vi "Upload Package to SLE.vi"(0 "PACKAGE_PATH":path, 5 "FEED_NAME":string, 11 "error in (no error)":errorcluster) -> (15 "error out":errorcluster)   [LabVIEW 2021, in "Measurement Builder.lvlib"]
uses:
  Measurement Builder.lvlib
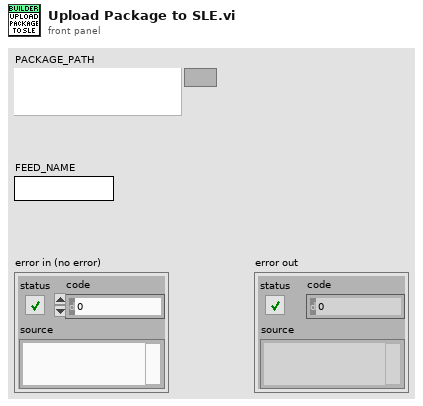
[diagram p1: front panel]
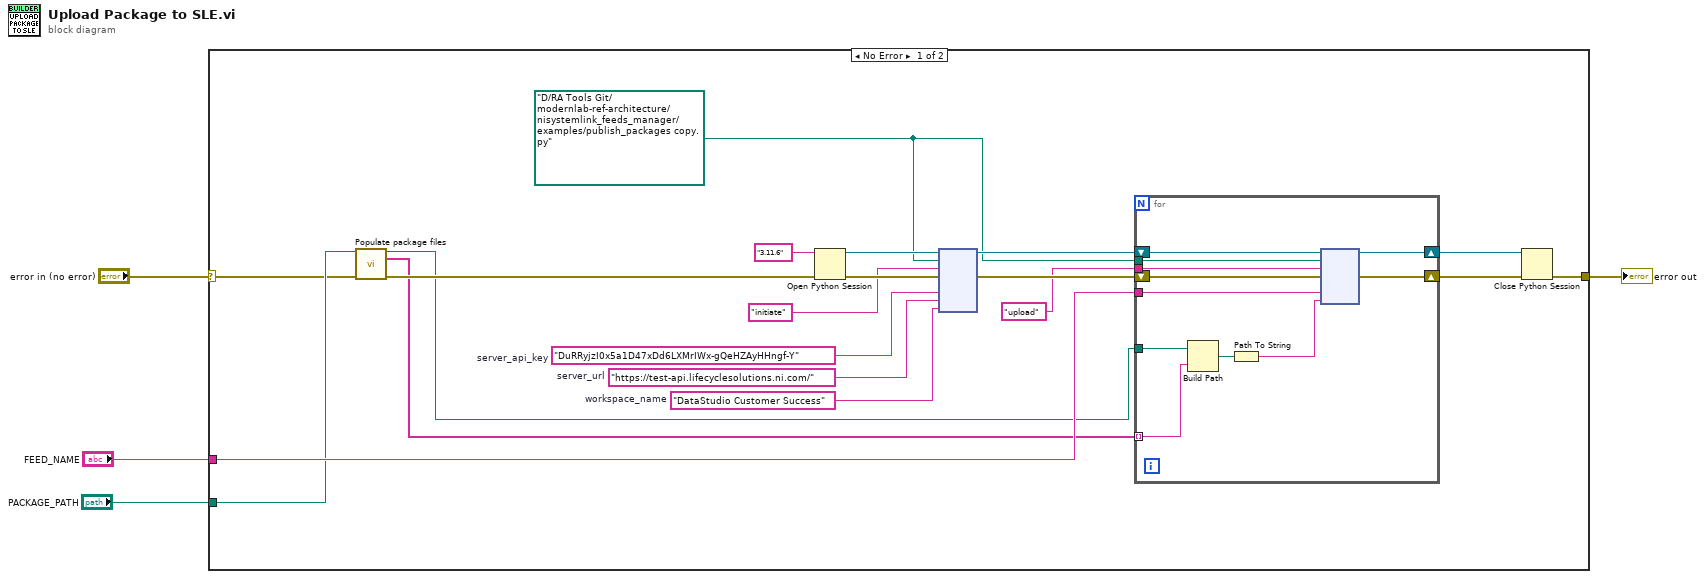
[diagram p0: block diagram]
diagram:
  n1 = case shown="No Error" "error in (no error)" {
    selector: "error in (no error)" -> [w8 w36]
    tunnel: "FEED_NAME" -> [w11 _]
    tunnel: "PACKAGE_PATH" -> [w9 _]
    tunnel: [w10 w36] -> w1
    frame No Error {
      w18 = "DataStudio Customer Success"  # workspace_name
      w19 = "https://test-api.lifecyclesolutions.ni.com/"  # server_url
      w20 = "DuRRyjzI0x5a1D47xDd6LXMrIWx-gQeHZAyHHngf-Y"  # server_api_key
      w12 = path "D:/RA Tools Git/modernlab-ref-architecture/nisystemlink_feeds_manager/examples/publish_packages copy.py" ("module path")
      n2 = call "Populate package files.vi"("Packages Path"=w9, "error in (no error)"=w8) -> ("path out"=w6:path, "filenames"=w5:string[], "error out"=w7:errorcluster)  [unwired: 11 in]
      n3 = Open Python Session(python version="3.11.6" ("Python version"), 3:w7) -> (session out=w23:refnum<k35>, error out=w22:errorcluster)  [unwired: 1 in]
      n4 = node(w23, w12, "initiate" ("function name"), w22, w20, w19, w18) -> (w17:refnum<k35>, w15:errorcluster)  [unwired: 5 in, 2 out]
      n5 = for {
        tunnel: "upload" ("function name") -> [w31]
        tunnel: w12 -> [w30]
        tunnel: w11 -> [w29]
        shift-right: [w34] -> w16
        shift-left: w17 -> [w35]
        shift-right: [w32] -> w14
        shift-left: w15 -> [w33]
        tunnel: w6 -> [w27]
        tunnel: w5 -> [w28] mode=indexing
        n6 = Build Path(base path=w27, name or relative path=w28) -> (appended path=w26:path)
        n7 = Path To String(path=w26) -> (string=w25:string)
        n8 = node(w35, w30, w31, w33, w29, w25) -> (w34:refnum<k35>, w32:errorcluster)  [unwired: 4 in, 2 out]
      }
      n9 = Close Python Session(session in=w16, error in=w14) -> (11:w10:errorcluster)
    }
    frame Error {
    }
  }
  "error out" <- w1
